vi "Color Sensor V3 Open.vi"(8 "error in (no error)":errorcluster, 10 "I2C Bus":T3=enum."Invalid") -> (0 "error out":errorcluster, 3 "ColorSensorDevRef":T1={"I2CDevRef"={"DevStatus"={"status"=FALSE, "code"=0, "source"=""}, "Device Address"=0, "Handle"=0, "I2C Bus"=enum."Invalid"}} {"I2CDevRef"."Device Address" format="%.0x"})   [LabVIEW 2023]
uses:
  <vilib>/Rock Robotics/SystemInterfaces/i2clib/i2c_bus.ctl
  Typedef/Color Sensor V3 DevRef.ctl
  <vilib>/Rock Robotics/WPI/I2C/WPI_I2CDevRef.ctl
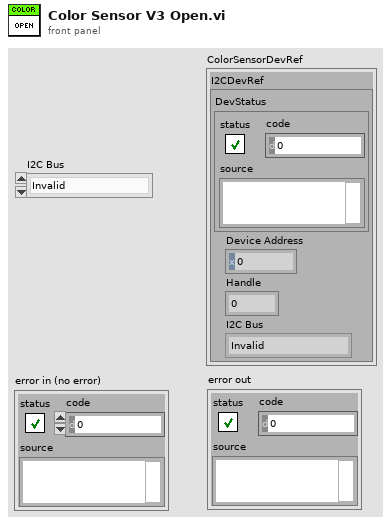
[diagram p1: front panel]
types:
  T1 = typedef "Color Sensor V3 DevRef.ctl" = cluster{"I2CDevRef":T2}
  T2 = typedef "WPI_I2CDevRef.ctl" = cluster{"DevStatus":errorcluster, "Device Address":u8, "Handle":i32, "I2C Bus":T3}
  T3 = typedef "i2c_bus.ctl" = enum16{"I2C On-Board", "I2C MXP", "Invalid"}
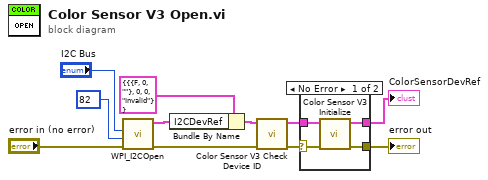
[diagram p0: block diagram]
diagram:
  n1 = call <vilib>:"WPI_I2COpen.vi"("error in"="error in (no error)", "Device Address"=u8 82, "I2C Bus"="I2C Bus") -> ("error out"=w3:errorcluster, "I2CDevRef"=w6:T2)  [unwired: 7 in]
  n2 = Bundle By Name(cluster=T1 {"I2CDevRef"={"DevStatus"={"status"=FALSE, "code"=0, "source"=""}, "Device Address"=0, "Handle"=0, "I2C Bus"=enum."Invalid"}} ("input cluster"), "I2CDevRef"=w6) -> (w4:T1)
  n3 = call "Color Sensor V3 Check Device ID.vi"("error in (no error)"=w3, "ColorSensorDevRef"=w4) -> ("error out"=w1:errorcluster, "ColorSensorDevRef out"=w2:T1)  [unwired: 8 in]
  n4 = case shown="No Error" w1 {
    selector: w1 -> [w12 w16]
    tunnel: w2 -> [w15 w17]
    tunnel: [w14 w17] -> w9
    tunnel: [w13 w16] -> w8
    frame No Error {
      n5 = call "Color Sensor V3 Initialize.vi"("error in (no error)"=w12, "ColorSensorDevRef"=w15) -> ("error out"=w13:errorcluster, "ColorSensorDevRef out"=w14:T1)  [unwired: 8 in]
    }
    frame Error {
    }
  }
  "ColorSensorDevRef" <- w9
  "error out" <- w8
